vi "Sort Array.vi"(11 "Sort Array":i8[](array[numeric])=[3, 9, 8, 11, 100, 14]) -> (3 "Sorted Array":i8[](array[numeric])=[3, -7, 8, -3, 100, 14])   [LabVIEW 2018]
panel:
  out "k":i32
  out "k+1":i32
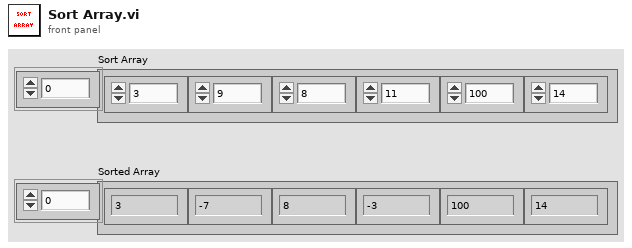
[diagram p1: front panel]
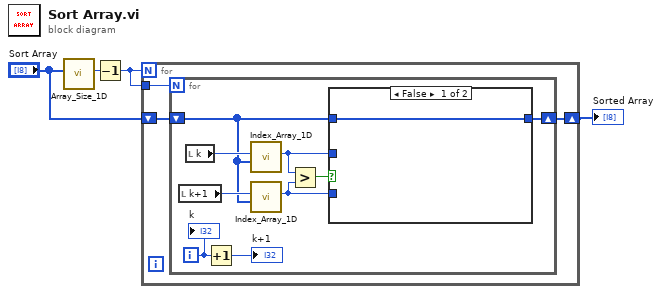
[diagram p0: block diagram]
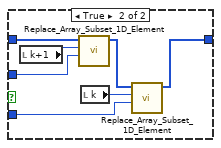
[diagram p2: hidden frame]
diagram:
  n1 = call "Array_Size_1D.vi"("Array"="Sort Array") -> ("Size"=w4:i32)  [unwired: 10 in]
  n2 = Decrement(x=w4) -> (x-1=w3:i32)
  n3 = for {
    N: w3 -> [_]
    tunnel: w3 -> [w7]
    shift-right: [w5] -> w1
    shift-left: "Sort Array" -> [w6]
    n4 = for {
      N: w7 -> [_]
      shift-right: [w8] -> w5
      shift-left: w6 -> [w11]
      i -> [w16]
      n5 = local read "k+1"() -> (w13:i32)
      n6 = local read "k"() -> (w14:i32)
      n7 = Increment(x=w16) -> (x+1=→"k+1":i32)
      n8 = call "Index_Array_1D.vi"("Index Array 1D"=w11, "Index"=w14) -> ("Value"=w10:i8)  [unwired: 9 in]
      n9 = call "Index_Array_1D.vi"("Index Array 1D"=w11, "Index"=w13) -> ("Value"=w9:i8)  [unwired: 9 in]
      n10 = Greater?(x=w10, y=w9) -> (0:w12:bool)
      n11 = case shown="False" w12 {
        tunnel: w11 -> [w17 w24]
        tunnel: w10 -> [_ w22]
        tunnel: w9 -> [_ w19]
        tunnel: [w17 w18] -> w8
        frame False {
        }
        frame True {
          n12 = local read "k+1"() -> (w23:i32)
          n13 = call "Replace_Array_Subset_1D_Element.vi"("Element RAS"=w22, "Index RAS1D"=w23, "RAS1D"=w24) -> ("New Array RAS1D"=w21:i8[])  [unwired: 8 in]
          n14 = local read "k"() -> (w20:i32)
          n15 = call "Replace_Array_Subset_1D_Element.vi"("Element RAS"=w19, "Index RAS1D"=w20, "RAS1D"=w21) -> ("New Array RAS1D"=w18:i8[])  [unwired: 8 in]
        }
      }
      "k" <- w16
    }
  }
  "Sorted Array" <- w1
